vi "Condition Indicator To Control.vi"(10 "Index":i32) -> (2 "Mapped Control Index":i32)   [LabVIEW 2025, in "_Msg Rescript.lvlib" / "_Msg Rescript.lvclass"]
uses:
  _Msg Rescript.lvclass
  _Msg Rescript.lvclass/_Msg Rescript.ctl
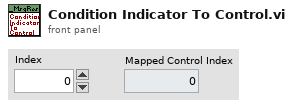
[diagram p1: front panel]
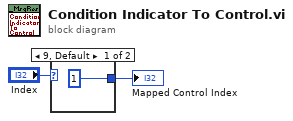
[diagram p0: block diagram]
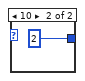
[diagram p2: hidden frame]
diagram:
  n1 = case shown="9, Default" "Index" {
    tunnel: [1 ("t") 2 ("t")] -> w1
    frame 9, Default {
    }
    frame 10 {
    }
  }
  "Mapped Control Index" <- w1
